vi "Read Joystick Buttons.vi"(8 "error in (no error)":errorcluster, 11 "LINX-SenseHat in":refnum<class "LINX-SenseHat.lvclass">) -> (0 "error out":errorcluster, 2 "Joystick Buttons":T1, 3 "LINX-SenseHat out":refnum<class "LINX-SenseHat.lvclass">)   [LabVIEW 2020, in "LINX-SenseHat.lvclass"]
uses:
  LINX-SenseHat.lvclass
  LINX-SenseHat.lvclass/LINX-SenseHat.ctl
  LINX I2C/LINX I2C.lvclass
  Joystick Buttons.ctl
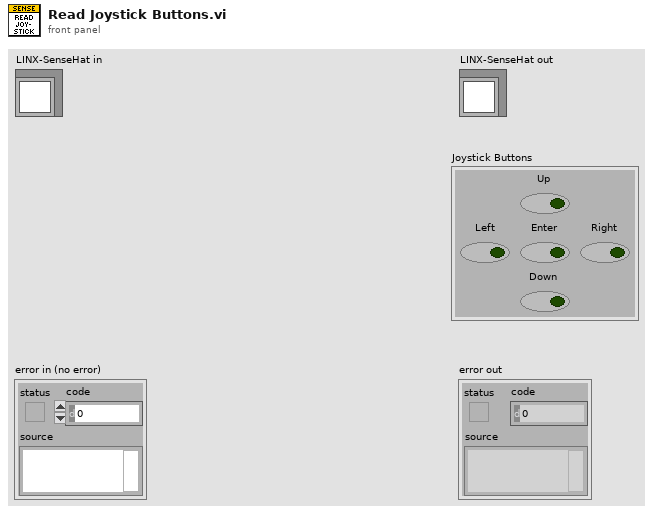
[diagram p1: front panel]
types:
  T1 = typedef "LINX-SenseHat.lvclass/Joystick Buttons.ctl" = cluster{"Down":bool, "Right":bool, "Up":bool, "Enter":bool, "Left":bool}
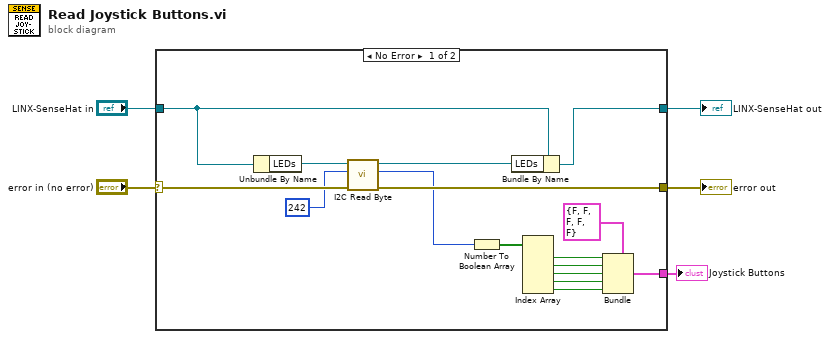
[diagram p0: block diagram]
diagram:
  n1 = case shown="No Error" "error in (no error)" {
    selector: "error in (no error)" -> [w17 w23]
    tunnel: [w16 w23] -> w4
    tunnel: [w18 w22] -> w2
    tunnel: "LINX-SenseHat in" -> [w19 w22]
    tunnel: [w6 _] -> w1
    frame No Error {
      n2 = Unbundle By Name(w19) -> ("LEDs"=w21:refnum<class "LINX I2C.lvclass">)
      n3 = call-dynamic "I2C Read Byte.vi"("error in (no error)"=w17, "Register Address"=u8 242, "LINX I2C in"=w21) -> ("error out"=w16:errorcluster, "Byte Read"=w14:u8, "LINX I2C out"=w20:refnum<class "LINX I2C.lvclass">)  [unwired: 6 in]
      n4 = Number To Boolean Array(number=w14) -> (Boolean array=w13:bool[])
      n5 = Bundle By Name(cluster=w19, "LEDs"=w20) -> (w18:refnum<class "LINX-SenseHat.lvclass">)
      n6 = Index Array(array=w13) -> (element #1=w12:bool, element #2=w11:bool, element #3=w10:bool, element #4=w9:bool, element #5=w8:bool)  [unwired: 5 in]
      n7 = Bundle(cluster=T1 {"Down"=FALSE, "Right"=FALSE, "Up"=FALSE, "Enter"=FALSE, "Left"=FALSE}, "Down"=w12, "Right"=w11, "Up"=w10, "Enter"=w9, "Left"=w8) -> (w6:T1)
    }
    frame Error {
    }
  }
  "error out" <- w4
  "LINX-SenseHat out" <- w2
  "Joystick Buttons" <- w1
